vi "Get IP Reg Types.vi"(10 "Version":T1, 11 "Analog Replay in":refnum<class "Analog Replay.lvclass">) -> (2 "IP Regs":variant[](array[variant]), 3 "Analog Replay out":refnum<class "Analog Replay.lvclass">)   [LabVIEW 2013, in "Analog Replay.lvclass"]
uses:
  Analog Replay.lvclass
  Bitfile Major Version.ctl
  Engine Simulation Session.lvclass
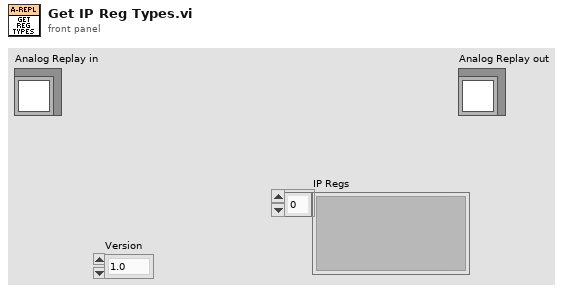
[diagram p1: front panel]
types:
  T1 = typedef "Engine Simulation Session.lvclass/Bitfile Major Version.ctl" = enum16{"1.0", "1.1", "1.2", "1.3"}
  T2 = cluster{"Data":i16[], "LoadOffset":u16, "Done":bool}
  T3 = cluster{"ReverseNegate":bool, "CycleAngle":bool, "SpeedThreshold":fxp<+/-,23,2>, "AOBelowThreshold":i16}
  T4 = cluster{"Offset":i16, "VScaleSlope":fxp<+,18,6>, "VScaleIntercept":fxp<+/-,18,3>}
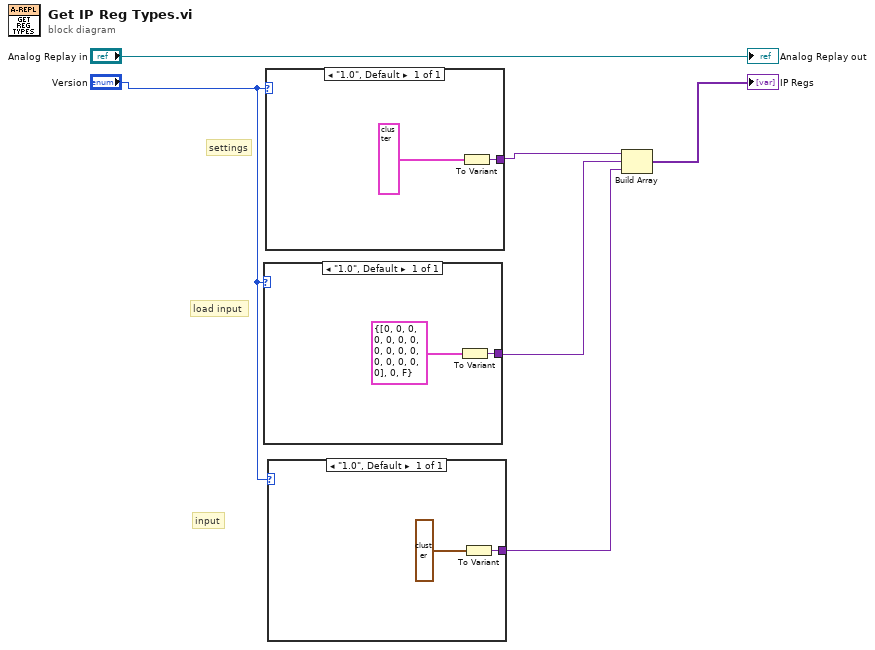
[diagram p0: block diagram]
diagram:
  # "input"
  # "load input"
  # "settings"
  n1 = case shown="\"1.0\", Default" "Version" {
    tunnel: [w8] -> w3
    frame "1.0", Default {
      n2 = To Variant(anything=T2 {"Data"=[0, 0, 0, 0, 0, 0, 0, 0, 0, 0, 0, 0, 0, 0, 0, 0], "LoadOffset"=0, "Done"=FALSE}) -> (Variant=w8:variant)
    }
  }
  n3 = case shown="\"1.0\", Default" "Version" {
    tunnel: [w10] -> w4
    frame "1.0", Default {
      n4 = To Variant(anything=T3 {"ReverseNegate"=FALSE, "CycleAngle"=FALSE, "SpeedThreshold"=0.0, "AOBelowThreshold"=0}) -> (Variant=w10:variant)
    }
  }
  n5 = case shown="\"1.0\", Default" "Version" {
    tunnel: [w12] -> w2
    frame "1.0", Default {
      n6 = To Variant(anything=T4 {"Offset"=0, "VScaleSlope"=0.0, "VScaleIntercept"=0.0}) -> (Variant=w12:variant)
    }
  }
  n7 = Build Array(w4, w3, w2) -> (→"IP Regs":variant[])
  "Analog Replay out" <- "Analog Replay in"
